vi "LIN_Process.vi"(10 "Data":T1={"Communication message"={"Sender"="", "receiver"="", "message"="", "data"=variant}, "LIN_Data"={"DLL_PATH"=path "", "Channels used"=1, "Funtiontype"=0, "Rx/TX"=enum."Rx", "Read message type"=enum."Receive&send messages", "async&sync"=enum."async", "sync_sendTimeout"=0, "LIN_SendHead"={"ALINIdxchn"=0, "ALINId"=0, "ALINDLC"=0}, "LIN_Set"={"Hardware Type"=2, "Hardware Subtype"=enum."TC1016", "AHwChannel"=0, "AAppChannel"=19, "ABaudrateKbps"=19.2, "AProtocol"=2, "AldHW"=0}, "LIN_DATA"={"Data0"=0, "Data1"=0, "Data2"=0, "Data3"=0, "Data4"=0, "Data5"=0, "Data6"=0, "Data7"=0}, "LIN_Set_Array"=[], "LDF"={"LDF Path"=path "", "LDF loading channel"=0}, "Blf_Log"={"Blf_Log_PATH"=path ""}, "LIN Scheduling Table Array"=[], "REC_Channel"=0}, "LIN Data array"=[], "error in"={"status"=FALSE, "code"=0, "source"=""}, "REC_Channel"=0, "AsynCall?"=FALSE, "DataBase_array"=refnum} {"REC_Channel" items=["CHN1", "CHN2", "CHN3", "CHN4", "CHN5", "CHN6", "CHN7", "CHN8", "CHN9", "CHN10", "CHN11", "CHN12", "CHN13", "CHN14", "CHN15", "CHN16", "CHN17", "CHN18", "CHN19", "CHN20", "CHN21", "CHN22", "CHN23", "CHN24", "CHN25", "CHN26", "CHN27", "CHN28", "CHN29", "CHN30", "CHN31", "CHN32"]; "LIN_Data"."REC_Channel" items=["CHN1", "CHN2", "CHN3", "CHN4", "CHN5", "CHN6", "CHN7", "CHN8", "CHN9", "CHN10", "CHN11", "CHN12", "CHN13", "CHN14", "CHN15", "CHN16", "CHN17", "CHN18", "CHN19", "CHN20", "CHN21", "CHN22", "CHN23", "CHN24", "CHN25", "CHN26", "CHN27", "CHN28", "CHN29", "CHN30", "CHN31", "CHN32"]; "LIN_Data"."LIN Scheduling Table Array"."LIN_Transmit"."Channel" items=["CHN1", "CHN2", "CHN3", "CHN4", "CHN5", "CHN6", "CHN7", "CHN8", "CHN9", "CHN10", "CHN11", "CHN12", "CHN13", "CHN14", "CHN15", "CHN16", "CHN17", "CHN18", "CHN19", "CHN20", "CHN21", "CHN22", "CHN23", "CHN24", "CHN25", "CHN26", "CHN27", "CHN28", "CHN29", "CHN30", "CHN31", "CHN32"]; "LIN_Data"."LIN Scheduling Table Array"."LIN_Transmit"."ID" format="%.0x"; "LIN_Data"."LIN Scheduling Table Array"."LIN_Transmit"."DLC" format="%.0x"; "LIN_Data"."LIN Scheduling Table Array"."LIN_Transmit"."Set_node_funtiontype" items=["MasterNode", "SlaveNode", "MonitorNote"]; "LIN_Data"."LDF"."LDF loading channel" items=["CHN1", "CHN2", "CHN3", "CHN4", "CHN5", "CHN6", "CHN7", "CHN8", "CHN9", "CHN10", "CHN11", "CHN12", "CHN13", "CHN14", "CHN15", "CHN16", "CHN17", "CHN18", "CHN19", "CHN20", "CHN21", "CHN22", "CHN23", "CHN24", "CHN25", "CHN26", "CHN27", "CHN28", "CHN29", "CHN30", "CHN31", "CHN32"]; "LIN_Data"."LIN_Set_Array"."Set_node_funtiontype" items=["MasterNode", "SlaveNode", "MonitorNote"]; "LIN_Data"."LIN_Set_Array"."Set"."Hardware Type" items=["BUS_UNKNOWN_TYPE", "TS_TCP_DEVICE", "XL_USB_DEVICE", "TS_USB_DEVICE", "PEAK_USB_DEVICE", "KVASER_USB_DEVICE", "ZLG_USB_DEVICE", "ICS_USB_DEVICE", "TS_TC1005_DEVICE", "CANABLE_USB_DEVICE", "TS_WIRELESS_OBD", "TS_USB_DEVICE_EX", "IXXAT_USB_DEVICE", "TS_ETH_IF_DEVICE", "TS_USB_IF_DEVICE", "BUS_DEV_TYPE_COUNT"]; "LIN_Data"."LIN_Set_Array"."Set"."AHwChannel" items=["CHN1", "CHN2", "CHN3", "CHN4", "CHN5", "CHN6", "CHN7", "CHN8", "CHN9", "CHN10", "CHN11", "CHN12", "CHN13", "CHN14", "CHN15", "CHN16", "CHN17", "CHN18", "CHN19", "CHN20", "CHN21", "CHN22", "CHN23", "CHN24", "CHN25", "CHN26", "CHN27", "CHN28", "CHN29", "CHN30", "CHN31", "CHN32"]; "LIN_Data"."LIN_Set_Array"."Set"."AAppChannel" items=["CHN1", "CHN2", "CHN3", "CHN4", "CHN5", "CHN6", "CHN7", "CHN8", "CHN9", "CHN10", "CHN11", "CHN12", "CHN13", "CHN14", "CHN15", "CHN16", "CHN17", "CHN18", "CHN19", "CHN20", "CHN21", "CHN22", "CHN23", "CHN24", "CHN25", "CHN26", "CHN27", "CHN28", "CHN29", "CHN30", "CHN31", "CHN32"]; "LIN_Data"."LIN_Set_Array"."Set"."AProtocol" items=["Lin_Protocol_13", "Lin_Protocol_20", "Lin_Protocol_21", "Lin_Protocol_J2602"]; "LIN_Data"."Funtiontype" items=["MasterNode", "SlaveNode", "MonitorNote"]; "LIN_Data"."LIN_SendHead"."ALINDLC" format="%.0x"; "LIN_Data"."LIN_SendHead"."ALINId" format="%.0x"; "LIN_Data"."LIN_SendHead"."ALINIdxchn" items=["CHN1", "CHN2", "CHN3", "CHN4", "CHN5", "CHN6", "CHN7", "CHN8", "CHN9", "CHN10", "CHN11", "CHN12", "CHN13", "CHN14", "CHN15", "CHN16", "CHN17", "CHN18", "CHN19", "CHN20", "CHN21", "CHN22", "CHN23", "CHN24", "CHN25", "CHN26", "CHN27", "CHN28", "CHN29", "CHN30", "CHN31", "CHN32"]; "LIN_Data"."LIN_Set"."Hardware Type" items=["BUS_UNKNOWN_TYPE", "TS_TCP_DEVICE", "XL_USB_DEVICE", "TS_USB_DEVICE", "PEAK_USB_DEVICE", "KVASER_USB_DEVICE", "ZLG_USB_DEVICE", "ICS_USB_DEVICE", "TS_TC1005_DEVICE", "CANABLE_USB_DEVICE", "TS_WIRELESS_OBD", "TS_USB_DEVICE_EX", "IXXAT_USB_DEVICE", "TS_ETH_IF_DEVICE", "TS_USB_IF_DEVICE", "BUS_DEV_TYPE_COUNT"]; "LIN_Data"."LIN_Set"."AHwChannel" items=["CHN1", "CHN2", "CHN3", "CHN4", "CHN5", "CHN6", "CHN7", "CHN8", "CHN9", "CHN10", "CHN11", "CHN12", "CHN13", "CHN14", "CHN15", "CHN16", "CHN17", "CHN18", "CHN19", "CHN20", "CHN21", "CHN22", "CHN23", "CHN24", "CHN25", "CHN26", "CHN27", "CHN28", "CHN29", "CHN30", "CHN31", "CHN32"]; "LIN_Data"."LIN_Set"."AAppChannel" items=["CHN1", "CHN2", "CHN3", "CHN4", "CHN5", "CHN6", "CHN7", "CHN8", "CHN9", "CHN10", "CHN11", "CHN12", "CHN13", "CHN14", "CHN15", "CHN16", "CHN17", "CHN18", "CHN19", "CHN20", "CHN21", "CHN22", "CHN23", "CHN24", "CHN25", "CHN26", "CHN27", "CHN28", "CHN29", "CHN30", "CHN31", "CHN32"]; "LIN_Data"."LIN_Set"."AProtocol" items=["Lin_Protocol_13", "Lin_Protocol_20", "Lin_Protocol_21", "Lin_Protocol_J2602"]; "LIN_Data"."Channels used" items=["1 Channel"=1, "2 Channels"=2, "3 Channels"=3, "4 Channels"=4, "5 Channels"=5]}, 11 "Queue Name":string="Demo_0") -> ()   [LabVIEW 2014]
uses:
  Typedef/TSLIN_SetData.ctl
  Typedef/TSLIN_SendHead.ctl
  <vilib>/Utility/miscctls.llb/LVPointTypeDef.ctl
  Utilities/Typedef/Hardware_Subtype.ctl
  Typedef/TLibLIN.ctl
  Typedef/TSLIN_Transmit.ctl
  All_Control/Typedef/Hardware Type.ctl
  Typedef/TSLIN_Config.ctl
  Typedef/TSLIN_Data.ctl
  Typedef/TSLIN_LIN Schedule_Table.ctl
  Typedef/TSLIN_LIN_Set.ctl
  All_Control/Typedef/Blf_Log.ctl
  DataBase/Typedef/CAN/TCANSignal.ctl
  DataBase/Typedef/LIN/TLINSignal.ctl
  DataBase/Typedef/FlexRay/TFlexRaySignal.ctl
  DataBase/Typedef/TDBSignalProperties.ctl
  DataBase/Typedef/TDBFrameProperties.ctl
  DataBase/Typedef/TDBECUProperties.ctl
  DataBase/Typedef/TDBProperties.ctl
  DataBase/Typedef/DataBase_array.ctl
  DataBase/Typedef/DataBase_array_index.ctl
panel:
  out "return":i32
  out "Set-data":bool
  out "loop value":i32
  in  "Channels used":u16(ring)=1 items=["1 Channel"=1, "2 Channels"=2, "3 Channels"=3, "4 Channels"=4, "5 Channels"=5, "6 Channels"=6, "7 Channels"=7, "8 Channels"=8, "9 Channels"=9, "10 Channels"=10, "11 Channels"=11, "12 Channels"=12, "13 Channels"=13, "14 Channels"=14, "15 Channels"=15, "16 Channels"=16]
  out "Receive Status":bool
  in  "Import":bool
  in  "Export":bool
  in  "Read Message Type":T13(ring)=enum."Receive&send messages"
  in  "LIN_DATA":T14 {"Data7" format="%x"; "Data6" format="%x"; "Data5" format="%x"; "Data4" format="%x"; "Data3" format="%x"; "Data2" format="%x"; "Data1" format="%x"; "Data0" format="%x"}
  in  "LIN_Data_0":i32(listbox)
  in  "Clear":bool
  in  "ALINDLC":u32 format="%.0x"
  in  "ALINId":u32 format="%.0x"
  in  "Rx/TX":enum16{"Rx", "Tx"}(ring)
  in  "Tag":T15(tab)
  in  "LIN_Schedule_Tab":bool
  in  "Cycle":bool=TRUE
  in  "SendHead&Receive":bool
  out "Successful ?":bool
  in  "ATimeoutMs":i32=200
  in  "Send_Frame":bool
  out "successful ？":bool
  in  "Cycle 2":bool=TRUE
  in  "async&sync":enum16{"async", "sync"}(ring)
  in  "Timeout":u16
  in  "Set_node_funtiontype":i32(ring) items=["MasterNode", "SlaveNode", "MonitorNote"]
  out "Setting ?":bool
  in  "Setting":bool
  in  "Config":bool
  in  "Hardware Subtype":T6=enum."TC1016"
  in  "AHwCh":i32(ring) items=["CHN1", "CHN2", "CHN3", "CHN4", "CHN5", "CHN6", "CHN7", "CHN8", "CHN9", "CHN10", "CHN11", "CHN12", "CHN13", "CHN14", "CHN15", "CHN16", "CHN17", "CHN18", "CHN19", "CHN20", "CHN21", "CHN22", "CHN23", "CHN24", "CHN25", "CHN26", "CHN27", "CHN28", "CHN29", "CHN30", "CHN31", "CHN32"]
  in  "AAppCh":i32(ring) items=["CHN1", "CHN2", "CHN3", "CHN4", "CHN5", "CHN6", "CHN7", "CHN8", "CHN9", "CHN10", "CHN11", "CHN12", "CHN13", "CHN14", "CHN15", "CHN16", "CHN17", "CHN18", "CHN19", "CHN20", "CHN21", "CHN22", "CHN23", "CHN24", "CHN25", "CHN26", "CHN27", "CHN28", "CHN29", "CHN30", "CHN31", "CHN32"]
  in  "Baudrate":sgl=19.2 format="%#_g  k"
  in  "Protocol":i32(ring)=2 items=["Lin_Protocol_13", "Lin_Protocol_20", "Lin_Protocol_21", "Lin_Protocol_J2602"]
  in  "DLL_PATH":path
  in  "STOP":bool
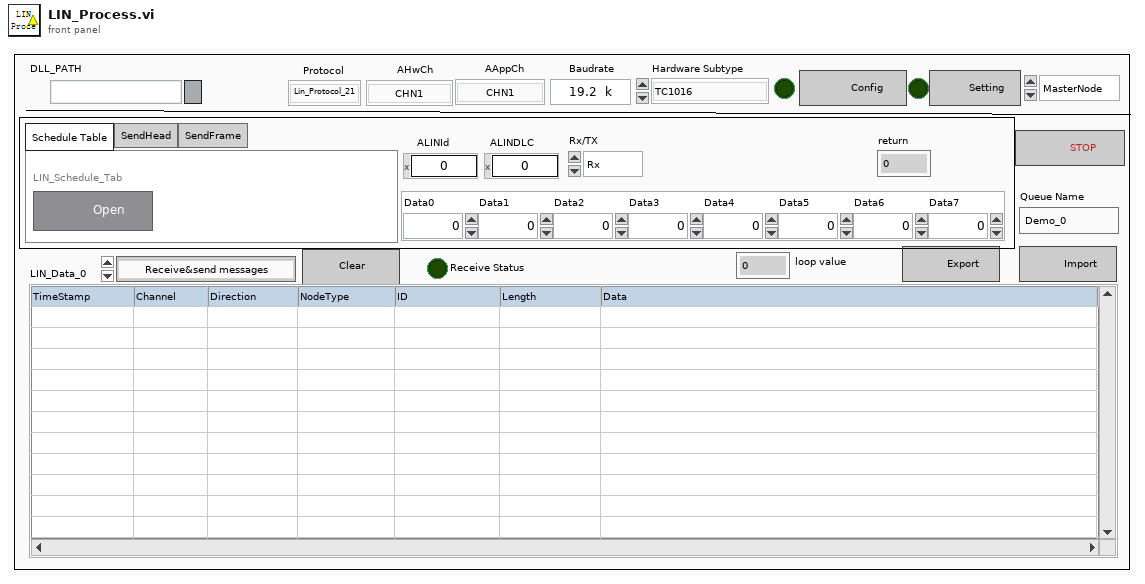
[diagram p1: front panel]
types:
  T1 = typedef "TSLIN_Data.ctl" = cluster{"Communication message":cluster{"Sender":string, "receiver":string, "message":string, "data":variant}, "LIN_Data":T2, "LIN Data array":T11[], "error in":errorcluster, "REC_Channel":i32, "AsynCall?":bool, "DataBase_array":T12}
  T2 = typedef "TSLIN_Config.ctl" = cluster{"DLL_PATH":path, "Channels used":u16, "Funtiontype":i32, "Rx/TX":enum16{"Rx", "Tx"}, "Read message type":enum16{"Only read received messages", "Receive&send messages"}, "async&sync":enum16{"async", "sync"}, "sync_sendTimeout":u16, "LIN_SendHead":T3, "LIN_Set":T4, "LIN_DATA":cluster{"Data0":u8, "Data1":u8, "Data2":u8, "Data3":u8, "Data4":u8, "Data5":u8, "Data6":u8, "Data7":u8}, "LIN_Set_Array":T7[], "LDF":cluster{"LDF Path":path, "LDF loading channel":i32}, "Blf_Log":T8, "LIN Scheduling Table Array":T9[], "REC_Channel":i32}
  T3 = typedef "TSLIN_SendHead.ctl" = cluster{"ALINIdxchn":u8, "ALINId":u32, "ALINDLC":u32}
  T4 = typedef "TSLIN_SetData.ctl" = cluster{"Hardware Type":T5, "Hardware Subtype":T6, "AHwChannel":i32, "AAppChannel":i32, "ABaudrateKbps":sgl, "AProtocol":i32, "AldHW":i32}
  T5 = typedef "Hardware Type.ctl" = i32
  T6 = typedef "Hardware_Subtype.ctl" = enum16{"TS_UNKNOWN_DEVICE", "TSCAN_PRO", "TSCAN_Lite1", "TC1001", "TL1001", "TC1011", "TM5011", "TC1002", "TC1014", "TSCANFD2517", "TC1026", "TC1016", "TC1012", "TC1013", "TLog1002", "TC1034", "TC1018", "GW2116", "TC2115", "MP1013", "TC1113", "TC1114", "TP1013", "TC1017", "TP1018", "TF10XX", "TL1004_FD_4_LIN_2", "TE1051", "TP1051", "TP1034", "TTS9015", "TP1026", "TTS1026", "TTS1034", "TTS1018", "TL1011", "TTS1015_LiAuto", "TTS1013_LiAuto", "TTS1016Pro", "TC1054Pro", "TC1054", "TLog1038", "TO1013", "TC1034Pro", "TC1018Pro", "TC1038Pro", "TS_DEV_END"}
  T7 = typedef "TSLIN_LIN_Set.ctl" = cluster{"Set":T4, "Set_node_funtiontype":i32}
  T8 = typedef "Blf_Log.ctl" = cluster{"Blf_Log_PATH":path}
  T9 = typedef "TSLIN_LIN Schedule_Table.ctl" = cluster{"LIN_Transmit":T10, "Delay(ms)":i32}
  T10 = typedef "TSLIN_Transmit.ctl" = cluster{"Channel":i32, "Rx/TX":enum16{"Rx", "Tx"}, "Set_node_funtiontype":i32, "DLC":u32, "ID":u32, "FDatas":cluster{"value0":u8, "value 1":u8, "value 2":u8, "value 3":u8, "value 4":u8, "value 5":u8, "value 6":u8, "value 7":u8}}
  T11 = typedef "TLibLIN.ctl" = cluster{"Ch":u8, "Code":u8, "Properties":u8, "FDLC":u8, "ID":u8, "Checksum":u8, "FStaus":u8, "FTimeUS":u64, "FDatas":cluster{"value0":u8, "value 1":u8, "value 2":u8, "value 3":u8, "value 4":u8, "value 5":u8, "value 6":u8, "value 7":u8}}
  T12 = typedef "DataBase_array_index.ctl" = refnum<vi>
  T13 = enum16{"Only read received messages", "Receive&send messages"}
  T14 = cluster{"Data0":u8, "Data1":u8, "Data2":u8, "Data3":u8, "Data4":u8, "Data5":u8, "Data6":u8, "Data7":u8}
  T15 = enum32{"Schedule Table", "SendHead", "SendFrame"}
  T16 = typedef "LVPointTypeDef.ctl" = cluster{"Horizontal":i16, "Vertical":i16}
  T17 = enum8{"Enabled", "Disabled", "Disabled and Grayed Out"}
  T18 = cluster{"Sender":string, "receiver":string, "message":string, "data":variant, "LIN Data array":T11[]}
  T19 = cluster{"Sender":string, "receiver":string, "message":string, "data":variant}
  T20 = enum32{"invalid app kind", "Development System", "Run Time System", "Student Edition", "Embedded LabVIEW", "Evaluation", "Custom"}
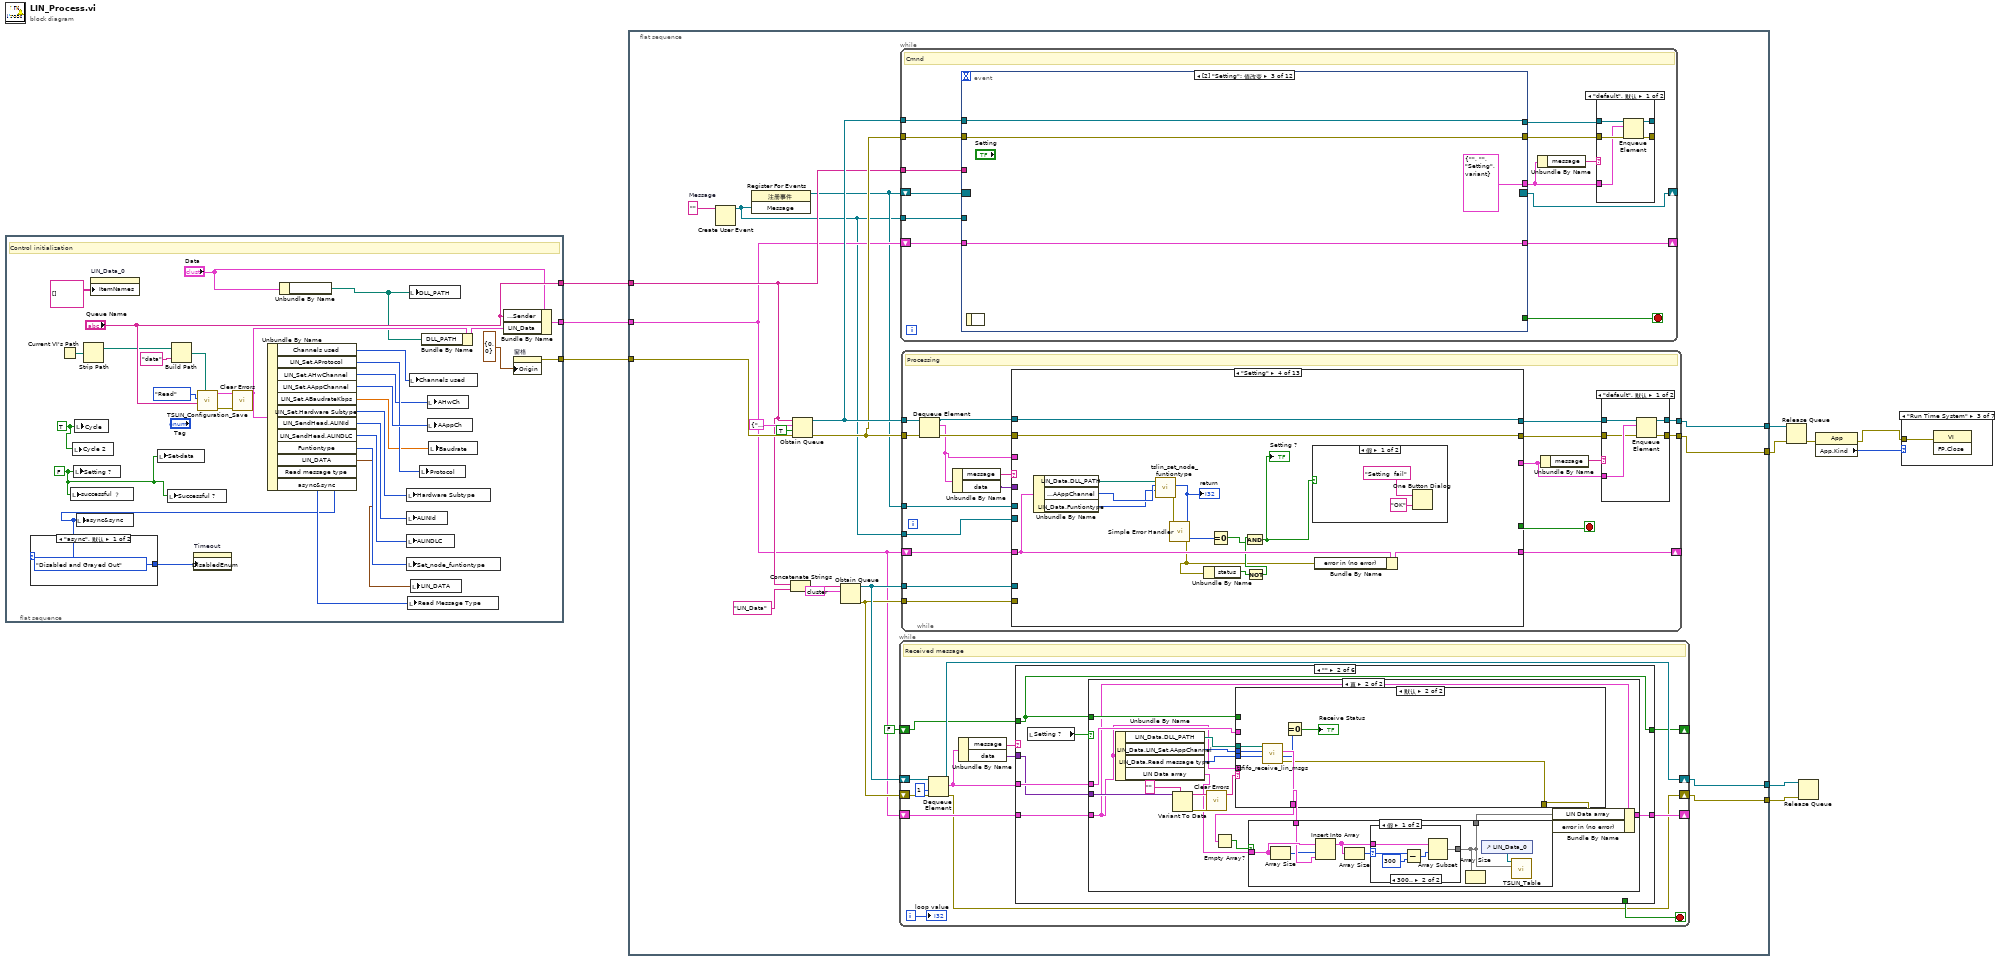
[diagram p0: block diagram]
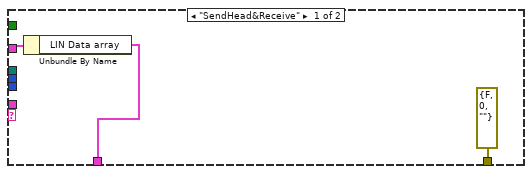
[diagram p6: hidden frame]
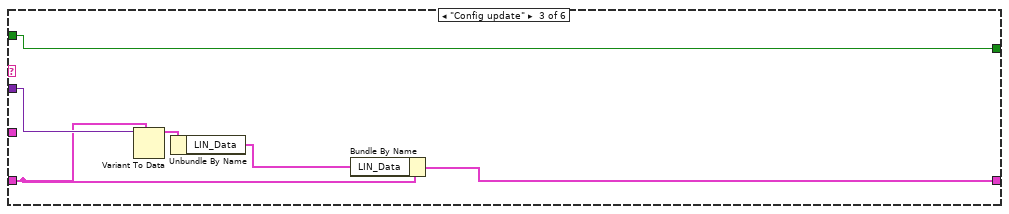
[diagram p7: hidden frame]
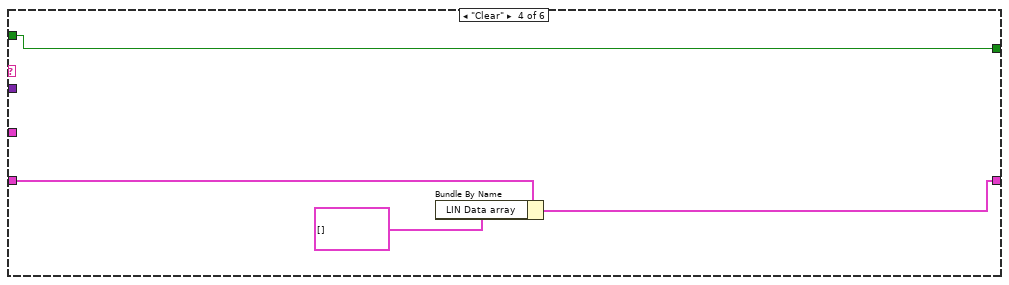
[diagram p8: hidden frame]
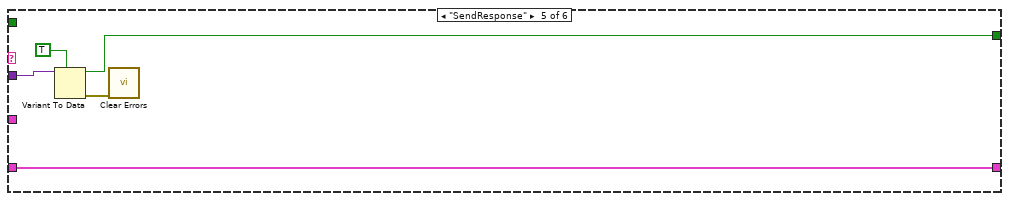
[diagram p9: hidden frame]
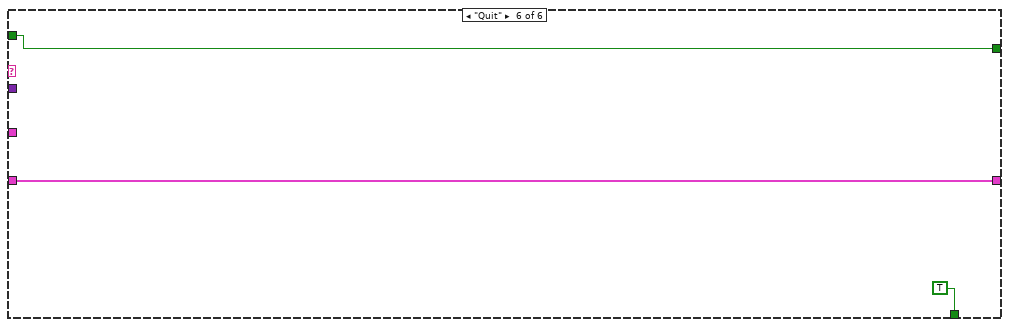
[diagram p10: hidden frame]
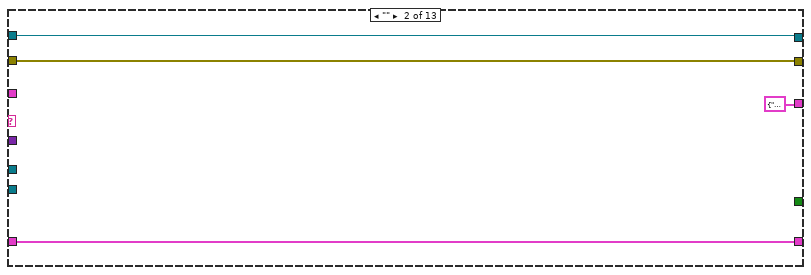
[diagram p13: hidden frame]
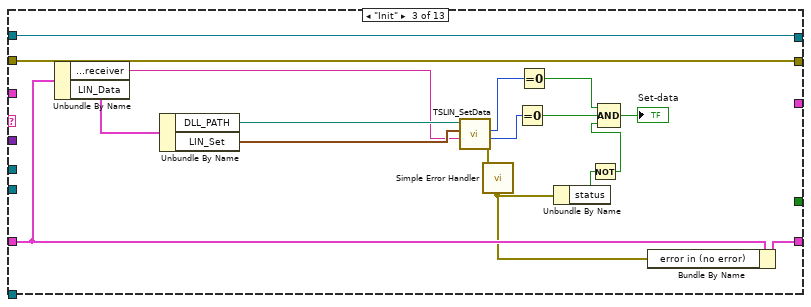
[diagram p14: hidden frame]
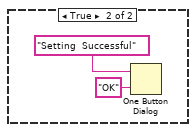
[diagram p15: hidden frame]
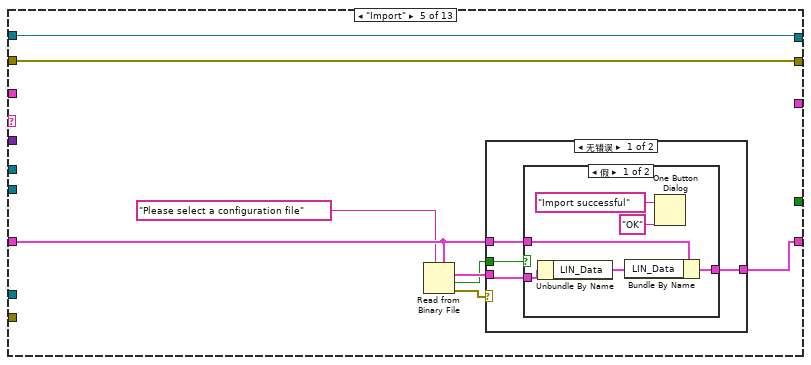
[diagram p16: hidden frame]
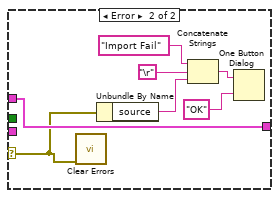
[diagram p18: hidden frame]
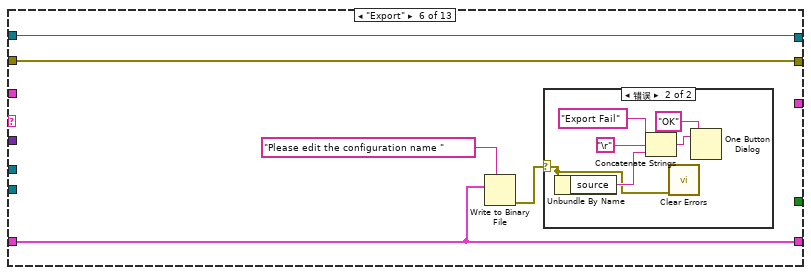
[diagram p19: hidden frame]
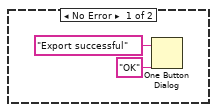
[diagram p20: hidden frame]
diagram:
  n1 = flat-sequence {
    tunnel: [w33] -> w10
    tunnel: ["Queue Name"] -> w9
    tunnel: [w28] -> w8
    frame #0 {
      w25 = TRUE ("Cycle")
      w14 = FALSE ("Connect ?")
      # "Control initialization"
      n2 = Current VI's Path() -> (path=w20:path)
      n3 = local write "successful ？"(w14) -> ()
      n4 = local write "Cycle 2"(w25) -> ()
      n5 = local write "Setting ?"(w14) -> ()
      n6 = local write "Cycle"(w25) -> ()
      n7 = Strip Path(path=w20) -> (stripped path=w18:path)  [unwired: 1 out]
      n8 = property on="LIN_Data_0" class="MCListbox (严格)"("ItemNames"=string[][] [] ("项名")) -> ()  [unwired: 2 in, 2 out]
      n9 = local write "Set-data"(w14) -> ()
      n10 = local write "Successful ?"(w14) -> ()
      n11 = Build Path(base path=w18, name or relative path="data") -> (appended path=w17:path)
      n12 = call "TSLIN_Configuration_Save.vi"("path"=w17, "Config Name"="Queue Name", "Read/Write"=enum16{"Read", "Write"}."Read") -> ("error in (no error) 2"=w13:errorcluster, "LIN_Data out"=w34:T2)  [unwired: 6 in, 1 out]
      n13 = call <vilib>:"Clear Errors.vi"("error in (no error)"=w13) -> ()  [unwired: 5 in, 2 out]
      n14 = Unbundle By Name(w34) -> ("Channels used"=w15:u16, "LIN_Set.AProtocol"=w37:i32, "LIN_Set.AHwChannel"=w36:i32, "LIN_Set.AAppChannel"=w38:i32, "LIN_Set.ABaudrateKbps"=w35:sgl, "LIN_Set.Hardware Subtype"=w39:T6, "LIN_SendHead.ALINId"=w31:u32, "LIN_SendHead.ALINDLC"=w30:u32, "Funtiontype"=w29:i32, "LIN_DATA"=w27:T14, "Read message type"=w23:T13, "async&sync"=w22:enum16{"async", "sync"})
      n15 = case shown="\"async\", 默认" w22 {
        tunnel: [T17."Disabled and Grayed Out" ("禁用") T17."Enabled" ("禁用")] -> w24
        frame "async", Default {
        }
        frame "sync" {
        }
      }
      n16 = local write "async&sync"(w22) -> ()
      n17 = property on="Timeout" class="DigNum (严格)"("DisabledEnum"=w24) -> ()  [unwired: 2 in, 2 out]
      n18 = Unbundle By Name("Data") -> ("LIN_Data.DLL_PATH"=w11:path)
      n19 = local write "Hardware Subtype"(w39) -> ()
      n20 = local write "ALINId"(w31) -> ()
      n21 = local write "ALINDLC"(w30) -> ()
      n22 = local write "Set_node_funtiontype"(w29) -> ()
      n23 = local write "Read Message Type"(w23) -> ()
      n24 = local write "DLL_PATH"(w11) -> ()
      n25 = local write "Channels used"(w15) -> ()
      n26 = local write "LIN_DATA"(w27) -> ()
      n27 = local write "Protocol"(w37) -> ()
      n28 = Bundle By Name(cluster=w34, "DLL_PATH"=w11) -> (w12:T2)
      n29 = local write "AHwCh"(w36) -> ()
      n30 = local write "AAppCh"(w38) -> ()
      n31 = local write "Baudrate"(w35) -> ()
      n32 = Bundle By Name(cluster="Data", "Communication message.Sender"="Queue Name", "LIN_Data"=w12) -> (w28:T1)
      n33 = property on="窗格" class="Pane"("Origin"=T16 {"Horizontal"=0, "Vertical"=0} ("原点")) -> (error out=w33:errorcluster)  [unwired: 2 in, 1 out]
    }
  }
  n34 = flat-sequence {
    tunnel: w10 -> [w61]
    tunnel: w9 -> [w55]
    tunnel: w8 -> [w50]
    tunnel: [w46] -> w6
    tunnel: [w45] -> w5
    tunnel: [w44] -> w2
    tunnel: [w43] -> w1
    frame #0 {
      w62 = ""  # Message
      n35 = Create User Event(user event datatype=w62) -> (user event=w47:refnum<user-event>)  [unwired: 1 in, 1 out]
      n36 = register-events(w47) -> (reference out=w48:refnum<event-registration>)  [unwired: 2 in, 1 out]
      n37 = Concatenate Strings(w55, "LIN_Data" ("字符串")) -> (w54:string)
      n38 = Obtain Queue(name (unnamed)=w55, element data type=T19 {"Sender"="", "receiver"="", "message"="", "data"=variant} ("Communication message"), create if not found? (T)=TRUE ("如未找到则创建？(T)"), error in (no error)=w61) -> (queue out=w60:refnum<queue>, error out=w59:errorcluster)  [unwired: 1 in, 1 out]
      n39 = Obtain Queue(name (unnamed)=w54, element data type=T18 {"Sender"="", "receiver"="", "message"="", "data"=variant, "LIN Data array"=[]} ("Communication message")) -> (queue out=w52:refnum<queue>, error out=w51:errorcluster)  [unwired: 3 in, 1 out]
      n40 = while {
        shift-right: [w67] -> w44
        shift-left: w52 -> [w76]
        shift-right: [w66] -> w43
        shift-left: w51 -> [w74]
        shift-right: [w69] -> _
        shift-left: w50 -> [w70]
        shift-right: [w65] -> _
        shift-left: FALSE -> [w64]
        i -> [w63]
        stop <- w71 stop-if-true
        # "Received message"
        n41 = Dequeue Element(queue=w76, timeout in ms (-1)=1 ("超时毫秒(-1)"), error in (no error)=w74) -> (queue out=w67:refnum<queue>, element=w68:T18, error out=w66:errorcluster)  [unwired: 1 out]
        n42 = Unbundle By Name(w68) -> ("message"=w73:string, "data"=w72:variant)
        n43 = case shown="\"\"" w73 {
          tunnel: w72 -> [_ w80 w131 _ w138 _]
          tunnel: [_ _ _ _ _ TRUE] -> w71
          tunnel: w70 -> [w78 w83 w130 w134 w140 w142]
          tunnel: [w78 w82 w129 w133 w140 w142] -> w69
          tunnel: w68 -> [_ w81 _ _ _ _]
          tunnel: [w77 w79 w126 w132 w136 w141] -> w65
          tunnel: w64 -> [w77 w79 w126 w132 _ w141]
          frame "假", Default {
          }
          frame "" {
            n44 = local read "Setting ?"() -> (w84:bool)
            n45 = case shown="真" w84 {
              tunnel: w83 -> [w85 w87]
              tunnel: [w85 w98] -> w82
              tunnel: w81 -> [_ w96]
              tunnel: w80 -> [_ w95]
              tunnel: w79 -> [_ w88]
              frame False {
              }
              frame True {
                n46 = Unbundle By Name(w87) -> ("LIN_Data.DLL_PATH"=w101:path, "LIN_Data.LIN_Set.AAppChannel"=w100:i32, "LIN_Data.Read message type"=w99:T13, "LIN Data array"=w91:T11[])
                n47 = Variant To Data(type="", Variant=w95) -> (data=w93:string, error out=w92:errorcluster)  [unwired: 1 in]
                n48 = call <vilib>:"Clear Errors.vi"("error in (no error)"=w92) -> ()  [unwired: 5 in, 2 out]
                n49 = case shown="默认" w93 {
                  tunnel: w101 -> [_ w125]
                  tunnel: w100 -> [_ w124]
                  tunnel: w99 -> [_ w123]
                  tunnel: [w117 w122] -> w90
                  tunnel: w96 -> [w118 _]
                  tunnel: w88 -> [_ _]
                  tunnel: w87 -> [_ _]
                  tunnel: [errorcluster {"status"=FALSE, "code"=0, "source"=""} ("error out") w119] -> w86
                  frame "SendHead&Receive" {
                    n50 = Unbundle By Name(w118) -> ("LIN Data array"=w117:T11[])
                  }
                  frame Default {
                    n51 = call "tsfifo_receive_lin_msgs.vi"("Read message type"=w123, "AIdxChn"=w124, "路径输入"=w125) -> ("错误输出"=w119:errorcluster, "return"=w121:i32, "ALINBuffer"=w122:T11[])  [unwired: 5 in, 1 out]
                    n52 = Equal To 0?(x=w121) -> (x = 0?=→"Receive Status":bool)
                  }
                }
                n53 = Empty Array?(array=w90) -> (empty?=w89:bool)
                n54 = case shown="假" w89 {
                  tunnel: [w102 w115] -> w97
                  tunnel: w91 -> [w107 w115]
                  tunnel: w90 -> [w106 _]
                  frame False {
                    n55 = Array Size(array=w107) -> (size(s)=w103:i32)
                    n56 = Insert Into Array(array=w107, index=w103, new element=w106) -> (w104:T11[])
                    n57 = Array Size(array=w104) -> (size(s)=w105:i32)
                    n58 = case shown="300.." w105 {
                      selector: w105 -> [_ w114]
                      tunnel: [w109 w112] -> w102
                      tunnel: w104 -> [w109 w110]
                      frame 0, Default {
                      }
                      frame 300.. {
                        n59 = Subtract(x=w114, y=300) -> (x-y=w111:i32)
                        n60 = Array Subset(array=w110, index=w111) -> (w112:T11[])  [unwired: 1 in]
                      }
                    }
                    n61 = Array Size(array=w102) -> ()  [unwired: 1 out]
                    n62 = control-ref of="LIN_Data_0"() -> (w108:refnum<vi>)
                    n63 = call "TSLIN_Table.vi"("LIN_Buffer"=w102, "LIN_Data Ref"=w108) -> ()  [unwired: 9 in, 1 out]
                  }
                  frame True {
                  }
                }
                n64 = Bundle By Name(cluster=w87, "LIN Data array"=w97, "error in (no error)"=w86) -> (w98:T1)
              }
            }
          }
          frame "Config update" {
            n65 = Variant To Data(type=w130, Variant=w131) -> (data=w128:T1)  [unwired: 1 in, 1 out]
            n66 = Unbundle By Name(w128) -> ("LIN_Data"=w127:T2)
            n67 = Bundle By Name(cluster=w130, "LIN_Data"=w127) -> (w129:T1)
          }
          frame "Clear" {
            n68 = Bundle By Name(cluster=w134, "LIN Data array"=T11[] []) -> (w133:T1)
          }
          frame "SendResponse" {
            n69 = Variant To Data(type=TRUE, Variant=w138) -> (data=w136:bool, error out=w137:errorcluster)  [unwired: 1 in]
            n70 = call <vilib>:"Clear Errors.vi"("error in (no error)"=w137) -> ()  [unwired: 5 in, 2 out]
          }
          frame "Quit" {
          }
        }
        "loop value" <- w63
      }
      n71 = while {
        tunnel: w60 -> [w457]
        tunnel: w59 -> [w455]
        tunnel: w55 -> [w451]
        shift-right: [w448] -> _
        shift-left: w50 -> [w449]
        shift-right: [w447] -> _
        shift-left: w48 -> [w450]
        tunnel: w47 -> [w446]
        stop <- w458 stop-if-true
        # "Cmnd"
        n72 = event shown="[2] \"Setting\": 值改变" {
          selector: w450 -> [_ _ _ _ _ _ _ _ _ _ _ _]
          dyn-events: [_ _ _ _ _ _ _ _ _ _ _ _] -> w447
          timeout: _ -> [_ _ _ _ _ _ _ _ _ _ _ _]
          tunnel: [_ _ _ _ _ _ _ _ _ w553 w563 TRUE ("放弃？")] -> w458
          tunnel: w457 -> [w468 w475 w479 w488 w499 w507 w511 w540 w549 w556 w562 w567]
          tunnel: [w468 w475 w479 w488 w499 w507 w511 w540 w549 w556 w562 w567] -> w456
          tunnel: [_ w473 T19 {"Sender"="", "receiver"="", "message"="Setting", "data"=variant} ("Communication message") w484 w494 w502 T19 {"Sender"="", "receiver"="", "message"="Clear", "data"=variant} ("Communication message") w527 w544 T19 {"Sender"="", "receiver"="", "message"="eee", "data"=variant} ("Communication message") w558 T19 {"Sender"="", "receiver"="", "message"="Quit", "data"=variant} ("Communication message")] -> w453
          tunnel: [w467 w469 w478 w487 w498 w506 w510 w523 w548 w551 w560 w565] -> w454
          tunnel: w455 -> [w467 w469 w478 w487 w498 w506 w510 w523 w548 w551 w560 w565]
          tunnel: w451 -> [_ _ _ _ _ _ _ _ _ _ _ _]
          tunnel: w449 -> [w466 w470 w477 w486 w497 w505 w509 w539 w547 w552 w561 w566]
          tunnel: [w466 w470 w477 w486 w497 w505 w509 w526 w547 w552 w561 w566] -> w448
          tunnel: w446 -> [_ _ _ _ _ _ _ _ _ _ _ _]
          event Timeout {
            n73 = event-data() -> ()  [unwired: 1 in, 3 out]
          }
          event "Config": Value Change {
            n74 = event-data() -> ()  [unwired: 1 in, 1 out]
            n75 = To Variant(anything=w470) -> (Variant=w471:variant)
            n76 = Bundle By Name(cluster=T19 {"Sender"="", "receiver"="", "message"="", "data"=variant} ("Communication message"), "message"="Init", "data"=w471) -> (w473:T19)
          }
          event "Setting": Value Change {
            n77 = event-data() -> ()  [unwired: 1 in, 1 out]
          }
          event "SendHead&Receive": Value Change {
            # "点击后，若发送成功显示闪烁\nAfter clicking, if the sending is successful, it will flash"
            n78 = event-data() -> ()  [unwired: 1 in, 1 out]
            n79 = flat-sequence {
              frame #0 {
                n80 = local write "Successful ?"(FALSE ("Successful ?")) -> ()
              }
              frame #1 {
                n81 = Wait (ms)(milliseconds to wait=u32 50 ("等待时间（毫秒）")) -> ()  [unwired: 1 out]
              }
            }
            n82 = property on="Rx/TX" class="Enum (严格)"("Val(Sgnl)"=enum16{"Rx", "Tx"}."Rx" ("值(信号)")) -> ()  [unwired: 2 in, 2 out]
            n83 = To Variant(anything="Cycle") -> (Variant=w481:variant)
            n84 = Bundle By Name(cluster=T19 {"Sender"="", "receiver"="", "message"="SendHead&Receive", "data"=variant} ("Communication message"), "message"="SendHead&Receive", "data"=w481) -> (w484:T19)
          }
          event "Send_Frame": Value Change {
            # "点击后，若发送成功显示闪烁\nAfter clicking, if the sending is successful, it will flash"
            n85 = event-data() -> ()  [unwired: 1 in, 1 out]
            n86 = property on="Rx/TX" class="Enum (严格)"("Val(Sgnl)"=enum16{"Rx", "Tx"}."Tx" ("值(信号)")) -> ()  [unwired: 2 in, 2 out]
            n87 = flat-sequence {
              frame #0 {
                n88 = local write "successful ？"(FALSE ("successful ？")) -> ()
              }
              frame #1 {
                n89 = Wait (ms)(milliseconds to wait=u32 50 ("等待时间（毫秒）")) -> ()  [unwired: 1 out]
              }
            }
            n90 = To Variant(anything="Cycle 2") -> (Variant=w493:variant)
            n91 = Bundle By Name(cluster=T19 {"Sender"="", "receiver"="", "message"="SendHead&Receive", "data"=variant} ("Communication message"), "message"="Send_Frame", "data"=w493) -> (w494:T19)
          }
          event "LIN_Schedule_Tab": Value Change {
            n92 = event-data() -> ()  [unwired: 1 in, 1 out]
            n93 = Bundle By Name(cluster=T19 {"Sender"="", "receiver"="", "message"="SendHead&Receive", "data"=variant} ("Communication message"), "message"="LIN_Schedule_Tab") -> (w502:T19)
          }
          event "Clear": Value Change {
            n94 = event-data() -> ()  [unwired: 1 in, 1 out]
          }
          event "DLL_PATH", "Protocol", "Baudrate", "AAppCh", "AHwCh", "ALINId", "ALINDLC", "Set_node_funtiontype", "Rx/TX", "LIN_DATA", "Timeout", "async&sync", "Read Message Type": Value Change {
            w534 = 3 items=["BUS_UNKNOWN_TYPE", "TS_TCP_DEVICE", "XL_USB_DEVICE", "TS_USB_DEVICE", "PEAK_USB_DEVICE", "KVASER_USB_DEVICE", "ZLG_USB_DEVICE", "ICS_USB_DEVICE", "TS_TC1005_DEVICE"] ("硬件类型")
            n95 = event-data() -> ()  [unwired: 1 in, 1 out]
            n96 = Bundle By Name(cluster=T4 {"Hardware Type"=3, "Hardware Subtype"=enum."TC1026", "AHwChannel"=0, "AAppChannel"=0, "ABaudrateKbps"=19.2, "AProtocol"=2, "AldHW"=0} ("Set"), "Hardware Type"=w534, "Hardware Subtype"="Hardware Subtype", "AHwChannel"="AHwCh", "AAppChannel"="AAppCh", "ABaudrateKbps"="Baudrate", "AProtocol"="Protocol") -> (w533:T4)
            n97 = case shown="\"async\", 默认" "async&sync" {
              tunnel: [T17."Disabled and Grayed Out" ("禁用") T17."Enabled" ("禁用")] -> w517
              frame "async", Default {
              }
              frame "sync" {
              }
            }
            n98 = Bundle By Name(cluster=T3 {"ALINIdxchn"=0, "ALINId"=0, "ALINDLC"=0} ("LIN_Data.LIN_SendHead"), "ALINIdxchn"="AAppCh", "ALINId"="ALINId", "ALINDLC"="ALINDLC") -> (w531:T3)
            n99 = Bundle By Name(cluster=w539, "LIN_Data.DLL_PATH"="DLL_PATH", "LIN_Data.sync_sendTimeout"="Timeout", "LIN_Data.LIN_DATA"="LIN_DATA", "LIN_Data.Rx/TX"="Rx/TX", "LIN_Data.LIN_Set"=w533, "LIN_Data.LIN_SendHead"=w531, "LIN_Data.Funtiontype"="Set_node_funtiontype", "LIN_Data.Read message type"="Read Message Type", "LIN_Data.Channels used"="Channels used") -> (w526:T1)
            n100 = property on="Timeout" class="DigNum (严格)"("DisabledEnum"=w517) -> ()  [unwired: 2 in, 2 out]
            n101 = To Variant(anything=w526) -> (Variant=w525:variant)
            n102 = Bundle By Name(cluster=T19 {"Sender"="", "receiver"="", "message"="", "data"=variant} ("Communication message"), "message"="Config update", "data"=w525) -> (w527:T19)
          }
          event "Export", "Import": Value Change {
            n103 = event-data() -> ("CtlRef"=w546:refnum<vi>)  [unwired: 1 in]
            n104 = property class="Bool"(reference=w546) -> ("Label.Text"=w543:string)  [unwired: 1 in, 2 out]
            n105 = Bundle By Name(cluster=T19 {"Sender"="", "receiver"="", "message"="", "data"=variant} ("Communication message"), "message"=w543) -> (w544:T19)
          }
          event User Event {
            n106 = event-data() -> ("Message"=w555:string)  [unwired: 1 in]
            n107 = Equal?(x=w555, y="Quit") -> (x = y?=w553:bool)
          }
          event Panel Close? {
            w563 = TRUE ("放弃？")
            n108 = event-data() -> ()  [unwired: 1 in, 4 out]
            n109 = Bundle By Name(cluster=T19 {"Sender"="", "receiver"="", "message"="", "data"=variant} ("Communication message"), "message"="Quit") -> (w558:T19)
            n110 = event-data("Discard?"=w563) -> ()  [unwired: 1 in, 1 out]
          }
          event "STOP": Value Change {
            n111 = event-data() -> ()  [unwired: 1 in, 1 out]
          }
        }
        n112 = Unbundle By Name(w453) -> ("message"=w452:string)
        n113 = case shown="\"default\", 默认" w452 {
          tunnel: w456 -> [w463 w465]
          tunnel: w454 -> [w462 w464]
          tunnel: w453 -> [w459 _]
          tunnel: [w461 w465] -> _
          tunnel: [w460 w464] -> _
          frame "default", Default {
            n114 = Enqueue Element(queue=w463, element=w459, error in (no error)=w462) -> (queue out=w461:refnum<queue>, error out=w460:errorcluster)  [unwired: 1 in, 1 out]
          }
          frame "" {
          }
        }
      }
      n115 = while {
        tunnel: w60 -> [w163]
        tunnel: w59 -> [w162]
        tunnel: [w155] -> w46
        tunnel: [w154] -> w45
        shift-right: [w150] -> _
        shift-left: w50 -> [w151]
        tunnel: w48 -> [w149]
        tunnel: w52 -> [w146]
        tunnel: w51 -> [w145]
        tunnel: w47 -> [w144]
        stop <- w153 stop-if-true
        # "Processing"
        n116 = Dequeue Element(queue=w163, error in (no error)=w162) -> (queue out=w160:refnum<queue>, element=w148:T19, error out=w159:errorcluster)  [unwired: 1 in, 1 out]
        n117 = Unbundle By Name(w148) -> ("message"=w161:string, "data"=w156:variant)
        n118 = case shown="\"Setting\"" w161 {
          tunnel: [w173 w177 w194 w208 w220 w243 w267 w315 w376 w391 w406 w412 w438] -> w158
          tunnel: w160 -> [w173 w177 w194 w208 w220 w243 w268 w316 w376 w391 w406 w412 w438]
          tunnel: w159 -> [w172 w176 w189 w207 w219 w242 w266 w320 w374 w390 w405 w408 w437]
          tunnel: [w172 w176 w189 w207 w219 w242 w265 w314 w370 w390 w405 w407 w437] -> w157
          tunnel: w156 -> [_ _ _ _ _ _ w274 w317 _ w393 w403 _ _]
          tunnel: [_ _ _ _ _ _ _ _ _ _ _ _ TRUE] -> w153
          tunnel: [w171 w175 w188 w204 w218 w241 w279 w323 w373 w379 w404 w409 w433] -> w150
          tunnel: w151 -> [w171 w175 w190 w206 w214 w241 w280 w321 w375 w378 w404 w410 w435]
          tunnel: w149 -> [_ _ _ _ _ _ _ _ _ _ _ _ w421]
          tunnel: [_ T19 {"Sender"="", "receiver"="", "message"="", "data"=variant} ("Communication message") _ _ _ _ w272 w310 _ _ _ _ _] -> w147
          tunnel: w148 -> [_ _ _ _ _ _ _ _ _ _ _ _ _]
          tunnel: w146 -> [_ _ _ _ _ _ w260 _ w369 w386 w401 _ w430]
          tunnel: w145 -> [_ _ _ _ _ _ w259 _ w368 w385 w400 _ w429]
          tunnel: w144 -> [_ _ _ _ _ _ _ _ _ _ _ _ w420]
          frame "eee", Default {
          }
          frame "" {
          }
          frame "Init" {
            n119 = Unbundle By Name(w190) -> ("Communication message.receiver"=w184:string, "LIN_Data"=w193:T2)
            n120 = Unbundle By Name(w193) -> ("DLL_PATH"=w192:path, "LIN_Set"=w191:T4)
            n121 = call "TSLIN_SetData.vi"("AppName"=w184, "Set"=w191, "Path"=w192) -> ("Error out"=w185:errorcluster, "mapping_return"=w182:i32, "config_baud_return"=w183:i32)  [unwired: 5 in, 1 out]
            n122 = call <vilib>:"Simple Error Handler.vi"("error in (no error)"=w185) -> ("error out"=w178:errorcluster)  [unwired: 4 in, 4 out]
            n123 = Equal To 0?(x=w182) -> (x = 0?=w180:bool)
            n124 = Equal To 0?(x=w183) -> (x = 0?=w181:bool)
            n125 = Unbundle By Name(w178) -> ("status"=w187:bool)
            n126 = Not(x=w187) -> (.not. x?=w186:bool)
            n127 = Compound Arithmetic op=AND(w181, w180, w186) -> (→"Set-data":bool)
            n128 = Bundle By Name(cluster=w190, "error in (no error)"=w178) -> (w188:T1)
          }
          frame "Setting" {
            n129 = Unbundle By Name(w206) -> ("LIN_Data.DLL_PATH"=w205:path, "LIN_Data.LIN_Set.AAppChannel"=w199:i32, "LIN_Data.Funtiontype"=w198:i32)
            n130 = call "tslin_set_node_funtiontype.vi"("set_node_funtiontype"=w198, "AAppChannel"=w199, "path"=w205) -> ("错误输出"=w200:errorcluster, "return"=w197:i32)  [unwired: 6 in, 1 out]
            "return" <- w197
            n131 = call <vilib>:"Simple Error Handler.vi"("error in (no error)"=w200) -> ("error out"=w195:errorcluster)  [unwired: 4 in, 4 out]
            n132 = Unbundle By Name(w195) -> ("status"=w202:bool)
            n133 = Equal To 0?(x=w197) -> (x = 0?=w196:bool)
            n134 = Not(x=w202) -> (.not. x?=w201:bool)
            n135 = Compound Arithmetic op=AND(w201, w196) -> (w203:bool)
            "Setting ?" <- w203
            n136 = case shown="假" w203 {
              frame False {
                n137 = One Button Dialog(message="Setting  fail" ("消息"), button name ("OK")="OK" ("按钮名称（“确定”）")) -> ()  [unwired: 1 out]
              }
              frame True {
                n138 = One Button Dialog(message="Setting  Successful" ("消息"), button name ("OK")="OK" ("按钮名称（“确定”）")) -> ()  [unwired: 1 out]
              }
            }
            n139 = Bundle By Name(cluster=w206, "error in (no error)"=w195) -> (w204:T1)
          }
          frame "Import" {
            n140 = Read from Binary File(5:w214, 7:"Please select a configuration file" ("对话框窗口（打开现有文件）")) -> (0:w217:errorcluster, 1:w215:bool, 2:w216:T1)  [unwired: 4 in, 1 out]
            n141 = case shown="无错误" w217 {
              selector: w217 -> [_ w235]
              tunnel: w216 -> [w222 _]
              tunnel: w215 -> [w224 _]
              tunnel: w214 -> [w223 w238]
              tunnel: [w221 w238] -> w218
              frame No Error {
                n142 = case shown="假" w224 {
                  tunnel: w223 -> [w230 w231]
                  tunnel: w222 -> [w229 _]
                  tunnel: [w227 w231] -> w221
                  frame False {
                    n143 = Unbundle By Name(w229) -> ("LIN_Data"=w228:T2)
                    n144 = Bundle By Name(cluster=w230, "LIN_Data"=w228) -> (w227:T1)
                    n145 = One Button Dialog(message="Import successful" ("消息"), button name ("OK")="OK" ("按钮名称（“确定”）")) -> ()  [unwired: 1 out]
                  }
                  frame True {
                  }
                }
              }
              frame Error {
                n146 = call <vilib>:"Clear Errors.vi"("error in (no error)"=w235) -> ()  [unwired: 5 in, 2 out]
                n147 = Unbundle By Name(w235) -> ("source"=w236:string)
                n148 = Concatenate Strings("Import Fail" ("消息"), "\r", w236) -> (w233:string)
                n149 = One Button Dialog(message=w233, button name ("OK")="OK" ("按钮名称（“确定”）")) -> ()  [unwired: 1 out]
              }
            }
          }
          frame "Export" {
            n150 = Write to Binary File(data=w241, 7:"Please edit the configuration name " ("提示（选择或输入文件路径）")) -> (error out=w239:errorcluster)  [unwired: 4 in, 2 out]
            n151 = case shown="错误" w239 {
              selector: w239 -> [_ w246]
              frame No Error {
                n152 = One Button Dialog(message="Export successful" ("消息"), button name ("OK")="OK" ("按钮名称（“确定”）")) -> ()  [unwired: 1 out]
              }
              frame Error {
                n153 = Unbundle By Name(w246) -> ("source"=w248:string)
                n154 = Concatenate Strings("Export Fail" ("消息"), "\r", w248) -> (w250:string)
                n155 = call <vilib>:"Clear Errors.vi"("error in (no error)"=w246) -> ()  [unwired: 5 in, 2 out]
                n156 = One Button Dialog(message=w250, button name ("OK")="OK" ("按钮名称（“确定”）")) -> ()  [unwired: 1 out]
              }
            }
          }
          frame "SendHead&Receive" {
            n157 = Variant To Data(type=FALSE, Variant=w274) -> (data=w270:bool, error out=w271:errorcluster)  [unwired: 1 in]
            n158 = case shown="无错误" w271 {
              selector: w271 -> [_ w296]
              tunnel: w270 -> [w281 _]
              tunnel: [w281 FALSE] -> w269
              tunnel: w268 -> [w285 w295]
              tunnel: w266 -> [w284 w294]
              tunnel: [w283 w293] -> w267
              tunnel: [w282 w292] -> w265
              frame No Error {
                n159 = case shown="假" w281 {
                  tunnel: w285 -> [w289 w291]
                  tunnel: w284 -> [w288 w290]
                  tunnel: [w287 w291] -> w283
                  tunnel: [w286 w290] -> w282
                  frame False {
                    n160 = Flush Queue(queue=w289, error in (no error)=w288) -> (queue out=w287:refnum<queue>, error out=w286:errorcluster)  [unwired: 1 out]
                  }
                  frame True {
                  }
                }
              }
              frame Error {
                n161 = call <vilib>:"Clear Errors.vi"("error in (no error)"=w296) -> ()  [unwired: 5 in, 2 out]
                n162 = Flush Queue(queue=w295, error in (no error)=w294) -> (queue out=w293:refnum<queue>, error out=w292:errorcluster)  [unwired: 1 out]
              }
            }
            n163 = Wait (ms)(milliseconds to wait=u32 10 ("等待时间（毫秒）")) -> ()  [unwired: 1 out]
            n164 = Unbundle By Name(w280) -> ("LIN_Data.DLL_PATH"=w278:path, "LIN_Data.LIN_SendHead.ALINIdxchn"=w261:u8, "LIN_Data.LIN_SendHead.ALINId"=w262:u32, "LIN_Data.LIN_SendHead.ALINDLC"=w277:u32)
            n165 = call "tsapp_transmit_header_and_receive_msg.vi"("ATimeoutMs"="ATimeoutMs", "ADLC"=w277, "AIdentifier"=w262, "AChn"=w261, "Path"=w278) -> ("错误输出"=w263:errorcluster, "return"=w264:i32, "ALINData"=w275:T11)  [unwired: 2 in, 1 out]
            n166 = Equal To 0?(x=w264) -> (x = 0?=→"Successful ?":bool)
            n167 = Build Array(w275) -> (w256:T11[])
            n168 = To Variant(anything="SendHead&Receive" ("Sender")) -> (Variant=w254:variant)
            n169 = Bundle By Name(cluster=T18 {"Sender"="", "receiver"="", "message"="", "data"=variant, "LIN Data array"=[]} ("Communication message"), "LIN Data array"=w256, "data"=w254) -> (w257:T18)
            n170 = Enqueue Element(queue=w260, element=w257, error in (no error)=w259) -> ()  [unwired: 1 in, 3 out]
            n171 = case shown="真" w269 {
              tunnel: [T19 {"Sender"="", "receiver"="", "message"="", "data"=variant} ("Communication message") w302] -> w272
              frame False {
              }
              frame True {
                n172 = To Variant(anything=TRUE) -> (Variant=w300:variant)
                n173 = Bundle By Name(cluster=T19 {"Sender"="", "receiver"="", "message"="", "data"=variant} ("Communication message"), "message"="SendHead&Receive", "data"=w300) -> (w302:T19)
              }
            }
            n174 = Bundle By Name(cluster=w280, "error in (no error)"=w263) -> (w279:T1)
          }
          frame "Send_Frame" {
            n175 = Unbundle By Name(w321) -> ("LIN_Data.async&sync"=w307:enum16{"async", "sync"}, "LIN_Data.sync_sendTimeout"=w308:u16, "LIN_Data.DLL_PATH"=w330:path, "LIN_Data.LIN_Set.AAppChannel"=w309:i32, "LIN_Data.Rx/TX"=w319:enum16{"Rx", "Tx"}, "LIN_Data.Funtiontype"=w327:i32, "LIN_Data.LIN_SendHead.ALINDLC"=w326:u32, "LIN_Data.LIN_SendHead.ALINId"=w325:u32, "LIN_Data.LIN_DATA"=w324:T14)
            n176 = Wait (ms)(milliseconds to wait=u32 10 ("等待时间（毫秒）")) -> ()  [unwired: 1 out]
            n177 = Variant To Data(type=FALSE, Variant=w317) -> (data=w313:bool, error out=w312:errorcluster)  [unwired: 1 in]
            n178 = Bundle By Name(cluster=T10 {"Channel"=0, "Rx/TX"=enum."Rx", "Set_node_funtiontype"=0, "DLC"=0, "ID"=0, "FDatas"={"value0"=0, "value 1"=0, "value 2"=0, "value 3"=0, "value 4"=0, "value 5"=0, "value 6"=0, "value 7"=0}} ("LIN_Transmit"), "Channel"=w309, "Rx/TX"=w319, "Set_node_funtiontype"=w327, "DLC"=w326, "ID"=w325, "FDatas"=w324) -> (w328:T10)
            n179 = case shown="\"async\", 默认" w307 {
              tunnel: w330 -> [w336 w341]
              tunnel: w328 -> [w335 w343]
              tunnel: [w334 w340] -> w322
              tunnel: [w333 w342] -> _
              tunnel: w320 -> [w332 w338]
              tunnel: [w331 w339] -> w306
              tunnel: w308 -> [_ w337]
              frame "async", Default {
                n180 = call "tsapp_transmit_lin_async.vi"("error in (no error)"=w332, "LIN_Transmit"=w335, "Path"=w336) -> ("error out"=w331:errorcluster, "return"=w334:i32, "Path output"=w333:path)  [unwired: 6 in]
              }
              frame "sync" {
                n181 = call "tsapp_transmit_lin_sync.vi"("错误输入（无错误）"=w338, "ATimeoutMS"=w337, "LIN_Transmit"=w343, "路径输入"=w341) -> ("错误输出"=w339:errorcluster, "return"=w340:i32, "路径输出"=w342:path)  [unwired: 5 in]
              }
            }
            n182 = Equal To 0?(x=w322) -> (x = 0?=→"successful ？":bool)
            n183 = case shown="无错误" w312 {
              selector: w312 -> [w350 w364]
              tunnel: w313 -> [w351 _]
              tunnel: [w351 FALSE] -> w311
              tunnel: w316 -> [w354 w363]
              tunnel: [w353 w362] -> w315
              tunnel: [w352 w361] -> w314
              frame No Error {
                n184 = case shown="假" w351 {
                  tunnel: w354 -> [w358 w360]
                  tunnel: [w357 w360] -> w353
                  tunnel: [w356 w359] -> w352
                  tunnel: w350 -> [w355 w359]
                  frame False {
                    n185 = Flush Queue(queue=w358, error in (no error)=w355) -> (queue out=w357:refnum<queue>, error out=w356:errorcluster)  [unwired: 1 out]
                  }
                  frame True {
                  }
                }
              }
              frame Error {
                n186 = call <vilib>:"Clear Errors.vi"("error in (no error)"=w364) -> ()  [unwired: 5 in, 2 out]
                n187 = Flush Queue(queue=w363) -> (queue out=w362:refnum<queue>, error out=w361:errorcluster)  [unwired: 1 in, 1 out]
              }
            }
            n188 = case shown="真" w311 {
              tunnel: [T19 {"Sender"="", "receiver"="", "message"="", "data"=variant} ("Communication message") w348] -> w310
              frame False {
              }
              frame True {
                n189 = To Variant(anything=TRUE) -> (Variant=w346:variant)
                n190 = Bundle By Name(cluster=T19 {"Sender"="", "receiver"="", "message"="", "data"=variant} ("Communication message"), "message"="Send_Frame", "data"=w346) -> (w348:T19)
              }
            }
            n191 = Bundle By Name(cluster=w321, "error in (no error)"=w306) -> (w323:T1)
          }
          frame "Clear" {
            w367 = T18 {"Sender"="", "receiver"="", "message"="", "data"=variant, "LIN Data array"=[]} ("Communication message")
            n192 = Bundle By Name(cluster=w367, "message"="Clear") -> ()  [unwired: 1 out]
            n193 = Enqueue Element(queue=w369, element=w367, error in (no error)=w368) -> ()  [unwired: 1 in, 3 out]
            n194 = property on="LIN_Data_0" class="MCListbox (严格)"(error in=w374, "ItemNames"=string[][] [] ("项名")) -> (error out=w370:errorcluster)  [unwired: 1 in, 1 out]
            n195 = Bundle By Name(cluster=w375, "LIN Data array"=T11[] []) -> (w373:T1)
          }
          frame "Config update" {
            n196 = Unbundle By Name(w378) -> ("Communication message.Sender"=w377:string)
            n197 = Variant To Data(type=w378, Variant=w393) -> (data=w392:T1, error out=w387:errorcluster)  [unwired: 1 in]
            n198 = Unbundle By Name(w392) -> ("LIN_Data"=w381:T2)
            n199 = Bundle By Name(cluster=w378, "LIN_Data"=w381) -> (w379:T1)
            n200 = To Variant(anything=w379) -> (Variant=w382:variant)
            n201 = Bundle By Name(cluster=T18 {"Sender"="", "receiver"="", "message"="", "data"=variant, "LIN Data array"=[]} ("Communication message"), "data"=w382, "message"="Config update") -> (w383:T18)
            n202 = call "TSLIN_Configuration_Save.vi"("error in (no error)"=w387, "Config Name"=w377, "Read/Write"=enum16{"Read", "Write"}."Write", "LIN_Data"=w381) -> ("error in (no error) 2"=w388:errorcluster)  [unwired: 5 in, 2 out]
            n203 = Bundle By Name(cluster=w379, "error in (no error)"=w388) -> ()  [unwired: 1 out]
            n204 = Enqueue Element(queue=w386, element=w383, error in (no error)=w385) -> ()  [unwired: 1 in, 3 out]
          }
          frame "SendResponse" {
            n205 = Variant To Data(type=TRUE, Variant=w403) -> (data=w398:bool, error out=w394:errorcluster)  [unwired: 1 in]
            n206 = To Variant(anything=w398) -> (Variant=w397:variant)
            n207 = call <vilib>:"Clear Errors.vi"("error in (no error)"=w394) -> ()  [unwired: 5 in, 2 out]
            n208 = Bundle By Name(cluster=T18 {"Sender"="", "receiver"="", "message"="", "data"=variant, "LIN Data array"=[]} ("Communication message"), "data"=w397, "message"="SendResponse") -> (w395:T18)
            n209 = Enqueue Element(queue=w401, element=w395, error in (no error)=w400) -> ()  [unwired: 1 in, 3 out]
          }
          frame "LIN_Schedule_Tab" {
            n210 = call "TSLIN_LIN_Schedule_Tab.vi"("错误输入（无错误）"=w408, "Data"=w410, "Sender"="LIN_Schedule_Tab") -> ("错误输出"=w407:errorcluster, "Data out"=w409:T1)  [unwired: 7 in]
          }
          frame "Quit" {
            n211 = Current VI's Path() -> (path=w425:path)
            n212 = Strip Path(path=w425) -> (stripped path=w415:path)  [unwired: 1 out]
            n213 = Bundle By Name(cluster=T18 {"Sender"="", "receiver"="", "message"="", "data"=variant, "LIN Data array"=[]} ("Communication message"), "message"="Quit") -> (w427:T18)
            n214 = Unbundle By Name(w435) -> ("LIN_Data.DLL_PATH"=w431:path, "LIN_Data"=w434:T2, "Communication message.Sender"=w424:string)
            n215 = Build Path(base path=w415, name or relative path="data") -> (appended path=w414:path)
            n216 = Enqueue Element(queue=w430, element=w427, error in (no error)=w429) -> ()  [unwired: 1 in, 3 out]
            n217 = call "TSLIN_Configuration_Save.vi"("path"=w414, "Config Name"=w424, "Read/Write"=enum16{"Read", "Write"}."Write", "LIN_Data"=w434) -> ("error in (no error) 2"=w432:errorcluster)  [unwired: 5 in, 2 out]
            n218 = disable-structure shown="启用" {
              disable-tunnel: w432 -> [w444 w445]
              disable-tunnel: w431 -> [w443 _]
              disable-tunnel: [w440 w445] -> w417
              frame Enabled {
                n219 = call "tsapp_disconnect.vi"("error in (no error)"=w444, "Path"=w443) -> ("error output"=w441:errorcluster, "Path output"=w442:path)  [unwired: 7 in, 1 out]
                n220 = call "finalize_lib_tsmaster.vi"("error in (no error)"=w441, "Path"=w442) -> ("error out"=w440:errorcluster)  [unwired: 8 in, 1 out]
              }
              frame Disabled {
              }
            }
            n221 = Generate User Event(user event=w420, event data cluster="Quit" ("y")) -> (user event out=w422:refnum<user-event>, error out=w418:errorcluster)  [unwired: 2 in]
            n222 = register-events(reference=w421, error in=w418, w422) -> (error out=w416:errorcluster)  [unwired: 1 out]
            n223 = Merge Errors(w417, w416) -> (w419:errorcluster)
            n224 = Bundle By Name(cluster=w435, "error in (no error)"=w419) -> (w433:T1)
          }
        }
        n225 = Unbundle By Name(w147) -> ("message"=w152:string)
        n226 = case shown="\"default\", 默认" w152 {
          tunnel: w158 -> [w168 w170]
          tunnel: w157 -> [w164 w169]
          tunnel: [w167 w170] -> w155
          tunnel: [w166 w169] -> w154
          tunnel: w147 -> [w165 _]
          frame "default", Default {
            n227 = Enqueue Element(queue=w168, element=w165, error in (no error)=w164) -> (queue out=w167:refnum<queue>, error out=w166:errorcluster)  [unwired: 1 in, 1 out]
          }
          frame "" {
          }
        }
      }
    }
  }
  n228 = Release Queue(queue=w6, error in (no error)=w5) -> (error out=w7:errorcluster)  [unwired: 1 in, 2 out]
  n229 = Release Queue(queue=w2, error in (no error)=w1) -> ()  [unwired: 1 in, 3 out]
  n230 = property class="App"(error in=w7) -> (error out=w4:errorcluster, "App.Kind"=w3:T20)  [unwired: 1 in, 1 out]
  n231 = case shown="\"Run Time System\"" w3 {
    tunnel: w4 -> [_ _ w569 _ _ _ _]
    frame "invalid app kind", Default {
    }
    frame "Development System" {
    }
    frame "Run Time System" {
      n232 = invoke class="VI" method="FP.Close"(error in=w569) -> ()  [unwired: 2 in, 3 out]
    }
    frame "Student Edition" {
    }
    frame "Embedded LabVIEW" {
    }
    frame "Evaluation" {
    }
    frame "Custom" {
    }
  }
